vi "Value to String.vi"(8 "error in":errorcluster, 11 "value":variant) -> (0 "error out":errorcluster, 2 "string":string, 3 "value dup":variant)   [LabVIEW 2020, in "Value.lvlib"]
uses:
  Value.lvlib
  Display Metadata.ctl
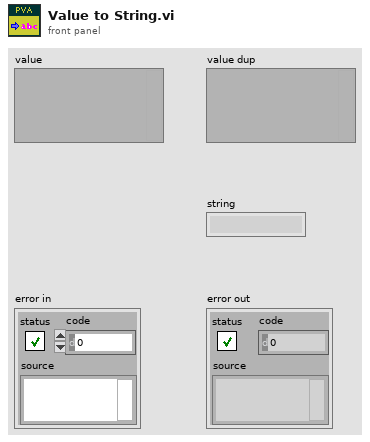
[diagram p1: front panel]
types:
  T1 = typedef "Value.lvlib/Display Metadata.ctl" = cluster{"Limit Low":dbl, "Limit High":dbl, "Description":string, "Units":string, "Precision":i32, "Form":enum32{"Default", "String", "Binary", "Decimal", "Hex", "Exponential", "Engineering"}}
  T2 = typedef "Value.lvlib/Type Code.ctl" = enum8{"Null", "Bool", "BoolA", "Int8", "Int8A", "Int16", "Int16A", "Int32", "Int32A", "Int64", "Int64A", "UInt8", "UInt8A", "UInt16", "UInt16A", "UInt32", "UInt32A", "UInt64", "UInt64A", "Float32", "Float32A", "Float64", "Float64A", "String", "StringA", "Struct", "StructA", "Union", "UnionA", "Any", "AnyA"}
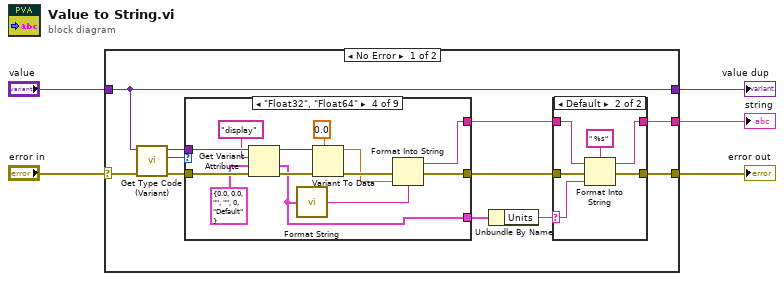
[diagram p0: block diagram]
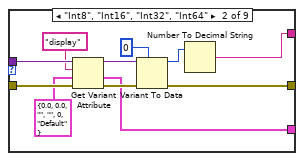
[diagram p4: hidden frame]
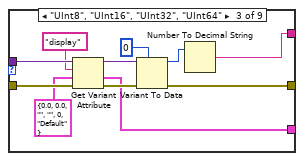
[diagram p5: hidden frame]
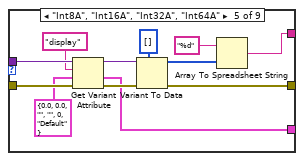
[diagram p6: hidden frame]
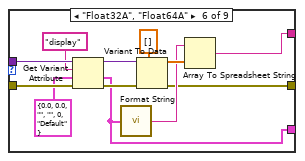
[diagram p7: hidden frame]
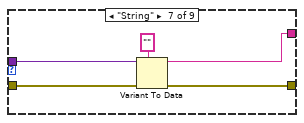
[diagram p8: hidden frame]
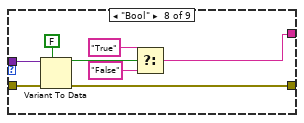
[diagram p9: hidden frame]
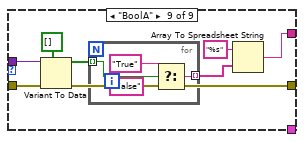
[diagram p10: hidden frame]
diagram:
  n1 = case shown="No Error" "error in" {
    selector: "error in" -> [w13 w111]
    tunnel: [w8 w111] -> w5
    tunnel: "value" -> [w12 w110]
    tunnel: [w12 w110] -> w2
    tunnel: [w6 _] -> w1
    frame No Error {
      n2 = call "Get Type Code (Variant).vi"("error in (no error)"=w13, "value"=w12) -> ("error out"=w16:errorcluster, "type code"=w15:T2, "value dup"=w14:variant)  [unwired: 5 in]
      n3 = case shown="\"Float32\", \"Float64\"" w15 {
        tunnel: w16 -> [w25 w32 w43 w53 w69 w81 w88 w96 w104]
        tunnel: w14 -> [_ w33 w44 w54 w70 w82 w89 w97 w105]
        tunnel: [w25 w26 w37 w58 w64 w74 w87 w95 w101] -> w9
        tunnel: [_ w28 w39 w49 w62 w73 w85 w90 w100] -> w7
        tunnel: [_ w29 w40 w48 w66 w76 _ _ _] -> w11
        frame Default {
        }
        frame "Int8", "Int16", "Int32", "Int64" {
          n4 = Get Variant Attribute(Variant=w33, name="display", default value (empty Variant)=T1 {"Limit Low"=0.0, "Limit High"=0.0, "Description"="", "Units"="", "Precision"=0, "Form"=enum."Default"} ("Display"), error in=w32) -> (duplicate Variant=w34:variant, value=w29:T1, error out=w35:errorcluster)  [unwired: 1 out]
          n5 = Variant To Data(error in=w35, type=i64 0, Variant=w34) -> (data=w27:i64, error out=w26:errorcluster)
          n6 = Number To Decimal String(number=w27) -> (decimal integer string=w28:string)  [unwired: 1 in]
        }
        frame "UInt8", "UInt16", "UInt32", "UInt64" {
          n7 = Get Variant Attribute(Variant=w44, name="display", default value (empty Variant)=T1 {"Limit Low"=0.0, "Limit High"=0.0, "Description"="", "Units"="", "Precision"=0, "Form"=enum."Default"} ("Display"), error in=w43) -> (duplicate Variant=w45:variant, value=w40:T1, error out=w46:errorcluster)  [unwired: 1 out]
          n8 = Variant To Data(error in=w46, type=u64 0, Variant=w45) -> (data=w38:u64, error out=w37:errorcluster)
          n9 = Number To Decimal String(number=w38) -> (decimal integer string=w39:string)  [unwired: 1 in]
        }
        frame "Float32", "Float64" {
          n10 = Get Variant Attribute(Variant=w54, name="display", default value (empty Variant)=T1 {"Limit Low"=0.0, "Limit High"=0.0, "Description"="", "Units"="", "Precision"=0, "Form"=enum."Default"} ("Display"), error in=w53) -> (duplicate Variant=w55:variant, value=w48:T1, error out=w56:errorcluster)  [unwired: 1 out]
          n11 = call "Format String.vi"("Display"=w48) -> ("format"=w50:string)
          n12 = Variant To Data(error in=w56, type=0.0, Variant=w55) -> (data=w57:dbl, error out=w59:errorcluster)
          n13 = Format Into String(format string=w50, error in=w59, w57) -> (resulting string=w49:string, error out=w58:errorcluster)  [unwired: 1 in]
        }
        frame "Int8A", "Int16A", "Int32A", "Int64A" {
          n14 = Get Variant Attribute(Variant=w70, name="display", default value (empty Variant)=T1 {"Limit Low"=0.0, "Limit High"=0.0, "Description"="", "Units"="", "Precision"=0, "Form"=enum."Default"} ("Display"), error in=w69) -> (duplicate Variant=w71:variant, value=w66:T1, error out=w72:errorcluster)  [unwired: 1 out]
          n15 = Variant To Data(error in=w72, type=i64[] [], Variant=w71) -> (data=w63:i64[], error out=w64:errorcluster)
          n16 = Array To Spreadsheet String(array=w63, 3:"%d" ("format string")) -> (spreadsheet string=w62:string)  [unwired: 1 in]
        }
        frame "Float32A", "Float64A" {
          n17 = Get Variant Attribute(Variant=w82, name="display", default value (empty Variant)=T1 {"Limit Low"=0.0, "Limit High"=0.0, "Description"="", "Units"="", "Precision"=0, "Form"=enum."Default"} ("Display"), error in=w81) -> (duplicate Variant=w83:variant, value=w76:T1, error out=w84:errorcluster)  [unwired: 1 out]
          n18 = call "Format String.vi"("Display"=w76) -> ("format"=w75:string)
          n19 = Variant To Data(error in=w84, type=dbl[] [], Variant=w83) -> (data=w77:dbl[], error out=w74:errorcluster)
          n20 = Array To Spreadsheet String(array=w77, 3:w75) -> (spreadsheet string=w73:string)  [unwired: 1 in]
        }
        frame "String" {
          n21 = Variant To Data(error in=w88, type="", Variant=w89) -> (data=w85:string, error out=w87:errorcluster)
        }
        frame "Bool" {
          n22 = Variant To Data(error in=w96, type=FALSE, Variant=w97) -> (data=w93:bool, error out=w95:errorcluster)
          n23 = Select(t="True", s=w93, f="False") -> (s? t:f=w90:string)
        }
        frame "BoolA" {
          n24 = Variant To Data(error in=w104, type=bool[] [], Variant=w105) -> (data=w102:bool[], error out=w101:errorcluster)
          n25 = for {
            tunnel: w102 -> [w107] mode=indexing
            tunnel: [w106] -> w99 mode=indexing
            n26 = Select(t="True", s=w107, f="False") -> (s? t:f=w106:string)
          }
          n27 = Array To Spreadsheet String(array=w99, 3:"%s" ("format string")) -> (spreadsheet string=w100:string)  [unwired: 1 in]
        }
      }
      n28 = Unbundle By Name(w11) -> ("Units"=w10:string)
      n29 = case shown="Default" w10 {
        selector: w10 -> [_ w19]
        tunnel: [w18 w23] -> w8
        tunnel: w9 -> [w18 w24]
        tunnel: w7 -> [w17 w21]
        tunnel: [w17 w20] -> w6
        frame "" {
        }
        frame Default {
          n30 = Format Into String(format string=" %s", initial string=w21, error in=w24, w19) -> (resulting string=w20:string, error out=w23:errorcluster)
        }
      }
    }
    frame Error {
    }
  }
  "error out" <- w5
  "string" <- w1
  "value dup" <- w2
